vi "PCC Test.vi"(8 "error in":errorcluster, 11 "IED Test in":refnum<class "IED Test.lvclass">) -> (0 "error out":errorcluster, 2 "Test Result":T1=enum."Success", 3 "IED Test out":refnum<class "IED Test.lvclass">)   [LabVIEW 2018, in "IED Test Framework.lvlib" / "IED Test.lvclass"]
uses:
  IED Test.lvclass
  C:/Program Files (x86)/National Instruments/LabVIEW 2018/vi.lib/ActorFramework/Actor/Actor.lvclass
  C:/Users/Administrator/Desktop/2018LabVIEW EMS/EMS Generic Actor/EMS Generic/EMS Generic.lvclass
  Controls/Test Result.ctl
  <vilib>/ORNL/CSEISMIC DDS/CSEISMIC DDS Base/Data Types/Controls/DeviceClass Selector.ctl
  PCC Actor/PCC/PCC.lvclass
  C:/Users/Administrator/Desktop/2018LabVIEW EMS/IED Actors/Device DDS Communications Framework/Device DDS Communications/Device DDS Communications.lvclass
  <vilib>/ActorFramework/Message Enqueuer/Message Enqueuer.lvclass/Message Enqueuer.ctl
  <vilib>/ActorFramework/Message Enqueuer/Enqueue.vi
  <vilib>/ActorFramework/Stop Msg/Stop Msg.lvclass
  C:/Program Files (x86)/National Instruments/LabVIEW 2018/vi.lib/ActorFramework/Message/Message.lvclass
  <vilib>/ActorFramework/Message Priority Queue/Priority Enqueue.vi
  Device DDS Communications Framework/Device DDS Communications/Device DDS Communications.lvclass
  <vilib>/ActorFramework/Actor/Actor.lvclass
  <vilib>/ORNL/CSEISMIC DDS/CSEISMIC DDS Base/CSEISMIC DDS.lvclass
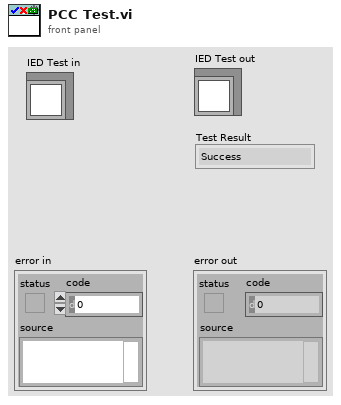
[diagram p1: front panel]
types:
  T1 = typedef "IED Test Framework.lvlib/IED Test.lvclass/Test Result.ctl" = enum16{"Invalid", "Success", "Failure", "Error", "Timeout"}
  T2 = typedef "CSEISMIC DDS.lvlib/CSEISMIC DDS.lvclass/DeviceClass Selector.ctl" = u16
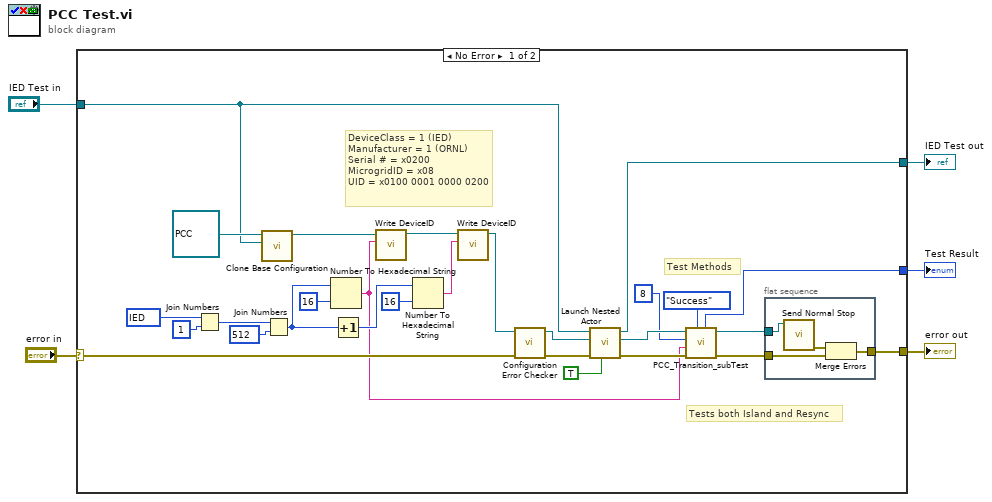
[diagram p0: block diagram]
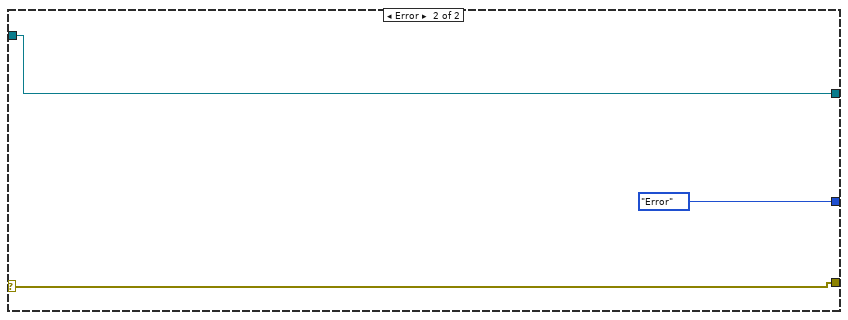
[diagram p2: hidden frame]
diagram:
  n1 = case shown="No Error" "error in" {
    selector: "error in" -> [w28 w40]
    tunnel: [w31 w40] -> w4
    tunnel: [w30 w39] -> w2
    tunnel: "IED Test in" -> [w7 w39]
    tunnel: [w23 Test_Result."Error" ("f")] -> w1
    frame No Error {
      w16 = T2 256 items=["Invalid"=0, "IED"=256, "DER"=512, "Relay"=768, "Meter"=1024, "Load"=1280, "Forecast"=1536, "Price"=1792, "Energy Storage"=513, "PV"=514, "Generator"=515, "Smart Relay"=769, "PCC"=770, "Smart Meter"=1025, "PMU"=1026, "HVAC"=1281] ("DeviceClass")
      # "DeviceClass = 1 (IED)\nManufacturer = 1 (ORNL)\nSerial # = x0200\nMicrogridID = x08\nUID = x0100 0001 0000 0200"
      # "Tests both Island and Resync"
      # "Test Methods"
      n2 = Join Numbers(hi=w16, lo=u16 1 ("MicrogridID")) -> ((hi.lo)=w13:u32)
      n3 = call-dynamic "Clone Base Configuration.vi"("Source Object"=w7, "Target Object in"=refnum<class "PCC.lvclass"> refnum ("PCC Actor.lvlib:PCC.lvclass")) -> ("Target Object out"=w6:refnum<class "PCC.lvclass">)  [unwired: 9 in]
      n4 = Join Numbers(hi=w13, lo=u32 512 ("MicrogridID")) -> ((hi.lo)=w18:u64)
      n5 = Number To Hexadecimal String(1:i16 16 ("width (-)"), 2:w18) -> (0:w9:string)
      n6 = Increment(x=w18) -> (x+1=w20:u64)
      n7 = call-dynamic "Write DeviceID.vi"("DeviceID"=w9, "Device DDS Communications in"=w6) -> ("Device DDS Communications out"=w15:refnum<class "PCC.lvclass">)  [unwired: 9 in]
      n8 = Number To Hexadecimal String(1:i16 16 ("width (-)"), 2:w20) -> (0:w21:string)
      n9 = call-dynamic "Write DeviceID.vi"("DeviceID"=w21, "Device DDS Communications in"=w15) -> ("Device DDS Communications out"=w11:refnum<class "PCC.lvclass">)  [unwired: 9 in]
      n10 = call "Configuration Error Checker.vi"("error in"=w28, "Device DDS Communications in"=w11) -> ("error out"=w32:errorcluster, "Device DDS Communications out"=w29:refnum<class "PCC.lvclass">)  [unwired: 8 in]
      n11 = call <vilib>:"Launch Nested Actor.vi"("Open Actor Core front panel? (F)"=TRUE, "error in (no error)"=w32, "Nested Actor"=w29, "Caller Actor in"=w7) -> ("error out"=w22:errorcluster, "Nested Actor's Enqueuer"=w27:refnum<class "Message Enqueuer.lvclass">, "Caller Actor out"=w30:refnum<class "IED Test.lvclass">)  [unwired: 5 in]
      n12 = call "PCC_Transition_subTest.vi"("Test Result in"=Test_Result."Success", "error in"=w22, "DeviceID"=w9, "MicrogridID"=u8 8, "Message Enqueuer in"=w27) -> ("error out"=w26:errorcluster, "Message Enqueuer out"=w24:refnum<class "Message Enqueuer.lvclass">, "Test Result out"=w23:T1)  [unwired: 2 in, 2 out]
      n13 = flat-sequence {
        tunnel: w24 -> [w37]
        tunnel: [w35] -> w31
        tunnel: w26 -> [w34]
        frame #0 {
          n14 = call <vilib>:"Send Normal Stop.vi"("Message Enqueuer"=w37) -> ("error out"=w36:errorcluster)  [unwired: 10 in]
          n15 = Merge Errors(w36, w34) -> (w35:errorcluster)
        }
      }
    }
    frame Error {
    }
  }
  "error out" <- w4
  "IED Test out" <- w2
  "Test Result" <- w1
